vi "recon.vi"(9 "N_det":dbl=40.0, 10 "N_rot":dbl=40.0, 11 "2-D Array of Real":dbl[][](array[numeric])) -> (0 "error out":errorcluster, 2 "Recon":T1(plugin-control))   [LabVIEW 2018]
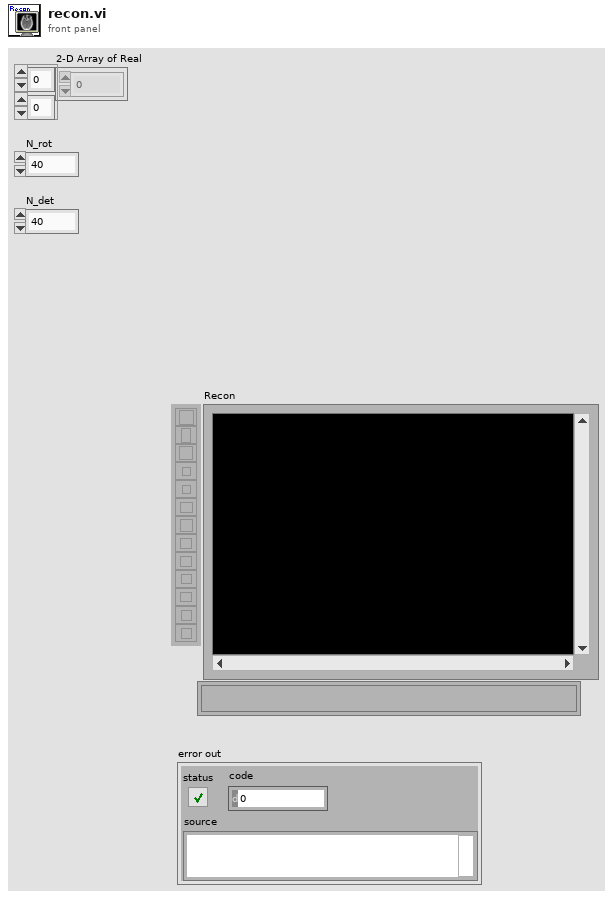
[diagram p1: front panel]
types:
  T1 = typedef "IMAQ Image.ctl" = refnum<image>
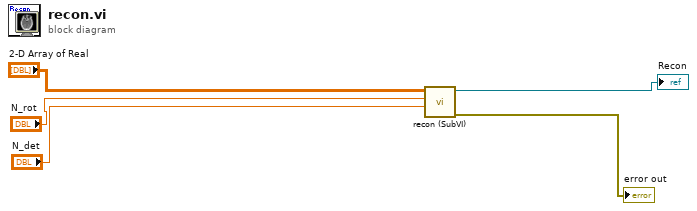
[diagram p0: block diagram]
diagram:
  n1 = call "recon (SubVI).vi"("N_det"="N_det", "N_rot"="N_rot", "2-D Array of Real"="2-D Array of Real") -> ("error out"=→"error out":errorcluster, "Refnum out"=→"Recon":T1)  [unwired: 7 in]
